vi "Generate Unique Header.vi"(8 "error in (no error)":errorcluster, 11 "PAS Data in":refnum<class "PAS Data.lvclass">) -> (0 "error out":errorcluster, 2 "Header":string[](array[string]), 3 "PAS Data out":refnum<class "PAS Data.lvclass">)   [LabVIEW 2014, in "PAS Library.lvlib" / "PAS Data.lvclass"]
uses:
  PAS Data.lvclass
  PAS Data.lvclass/PAS Data.ctl
  Data/Data.lvclass/Data.ctl
  Data/Read Data ID.vi
  Cell/PAS Cell Data.lvclass
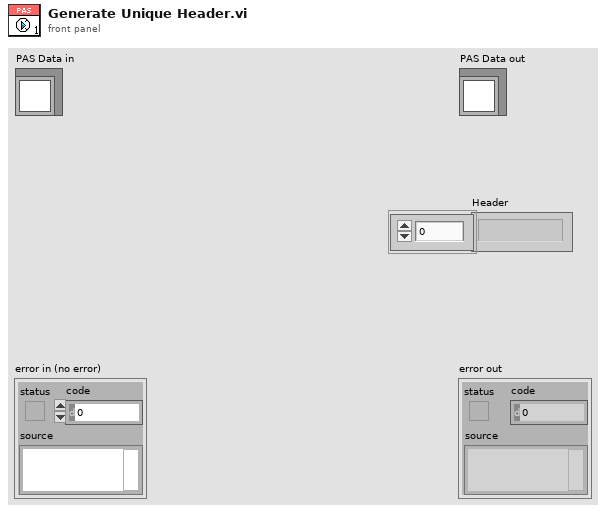
[diagram p1: front panel]
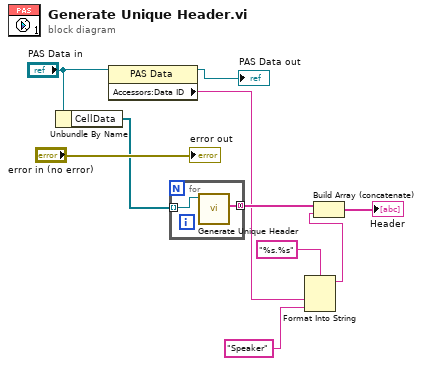
[diagram p0: block diagram]
diagram:
  n1 = Unbundle By Name("PAS Data in") -> ("CellData"=w9:refnum<class "PAS Cell Data.lvclass">[])
  n2 = property class="PAS Data"(reference="PAS Data in") -> (reference out=→"PAS Data out":refnum<class "PAS Data.lvclass">, "Accessors:Data ID"=w3:string)  [unwired: 1 in, 1 out]
  n3 = for {
    tunnel: w9 -> [w12] mode=indexing
    tunnel: [w11] -> w8 mode=concatenating
    n4 = call-dynamic "Generate Unique Header.vi"("PAS Cell Data in"=w12) -> ("Header"=w11:string[])  [unwired: 8 in, 2 out]
  }
  n5 = Format Into String(format string="%s.%s", w3, "Speaker") -> (resulting string=w1:string)  [unwired: 2 in, 1 out]
  n6 = Build Array (concatenate)(w8, w1) -> (→"Header":string[])
  "error out" <- "error in (no error)"
